vi "Draw_Pattern_exercise.vi"() -> ()   [LabVIEW 2016]
uses:
  Classes/Controller/Motion/A3200 Folder/A3200.lvclass
panel:
  out "XYZTheta Out 2":dbl[](array[numeric])
  out "XYZTheta Out":dbl[](array[numeric])
  in  "Speed":dbl
  in  "XY":dbl[](array[numeric])
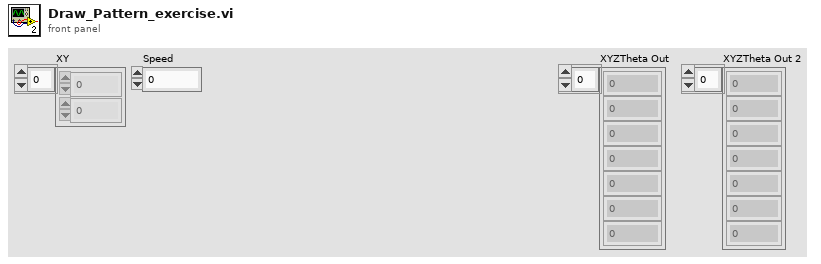
[diagram p1: front panel]
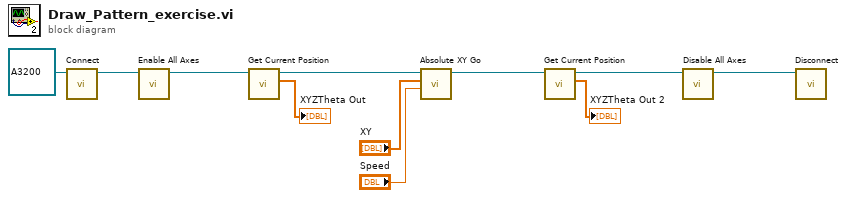
[diagram p0: block diagram]
diagram:
  n1 = call-dynamic "Connect.vi"("Gantry in"=refnum<class "A3200.lvclass"> refnum ("A3200.lvclass")) -> ("Gantry out"=w10:refnum<class "A3200.lvclass">)  [unwired: 9 in, 1 out]
  n2 = call-dynamic "Enable All Axes.vi"("A3200 in"=w10) -> ("A3200 out"=w6:refnum<class "A3200.lvclass">)  [unwired: 9 in, 1 out]
  n3 = call-dynamic "Get Current Position.vi"("Gantry in"=w6) -> ("XYZTheta Out"=→"XYZTheta Out":dbl[], "Gantry out"=w5:refnum<class "A3200.lvclass">)  [unwired: 8 in, 1 out]
  n4 = call-dynamic "Absolute XY Go.vi"("Speed"="Speed", "XY"="XY", "Gantry in"=w5) -> ("Gantry out"=w3:refnum<class "A3200.lvclass">)  [unwired: 7 in, 1 out]
  n5 = call-dynamic "Get Current Position.vi"("Gantry in"=w3) -> ("XYZTheta Out"=→"XYZTheta Out 2":dbl[], "Gantry out"=w2:refnum<class "A3200.lvclass">)  [unwired: 8 in, 1 out]
  n6 = call-dynamic "Disable All Axes.vi"("Gantry in"=w2) -> ("Gantry out"=w9:refnum<class "A3200.lvclass">)  [unwired: 9 in, 1 out]
  n7 = call-dynamic "Disconnect.vi"("Gantry in"=w9) -> ()  [unwired: 9 in, 1 out]
